vi "Ball Intake.vi"(9 "Scaling factor":dbl=0.5, 10 "Outtake":bool, 11 "Intake":bool) -> (3 "IntakeSpeed":dbl)   [LabVIEW 2018]
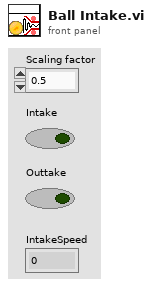
[diagram p1: front panel]
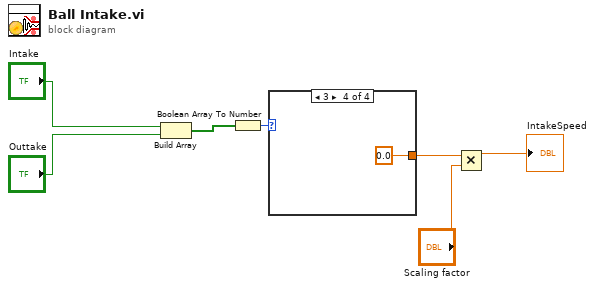
[diagram p0: block diagram]
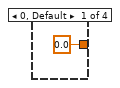
[diagram p2: hidden frame]
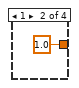
[diagram p3: hidden frame]
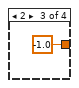
[diagram p4: hidden frame]
diagram:
  n1 = Build Array("Intake", "Outtake") -> (w5:bool[])
  n2 = Boolean Array To Number(Boolean array=w5) -> (number=w4:u32)
  n3 = case shown="3" w4 {
    tunnel: [0.0 1.0 -1.0 0.0] -> w3
    frame 0, Default {
    }
    frame 1 {
    }
    frame 2 {
    }
    frame 3 {
    }
  }
  n4 = Multiply(x=w3, y="Scaling factor") -> (x*y=→"IntakeSpeed":dbl)
